vi "PAN_sendSchedCmd.vi"(6 "timeout in ms (5000)":i32=5000, 8 "error in (no error)":errorcluster, 10 "command":string) -> (0 "error out":errorcluster, 2 "response":string)   [LabVIEW 2016]
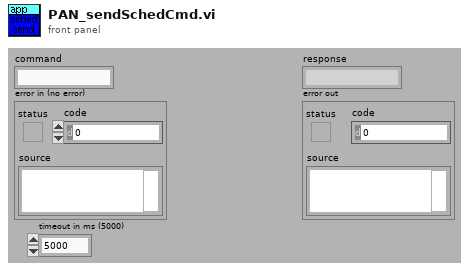
[diagram p1: front panel]
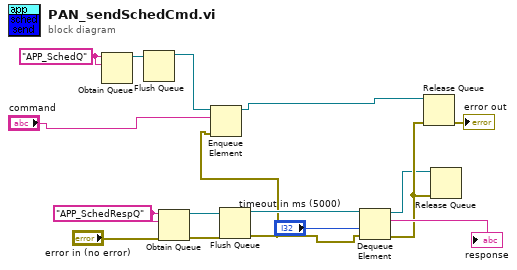
[diagram p0: block diagram]
diagram:
  w15 = "APP_SchedRespQ" ("name (unnamed)")
  w16 = "APP_SchedQ" ("name (unnamed)")
  n1 = Obtain Queue(name (unnamed)=w16, element data type=w16) -> (queue out=w10:refnum<queue>)  [unwired: 3 in, 2 out]
  n2 = Flush Queue(queue=w10) -> (queue out=w9:refnum<queue>)  [unwired: 1 in, 2 out]
  n3 = Obtain Queue(name (unnamed)=w15, element data type=w15, error in (no error)="error in (no error)") -> (queue out=w8:refnum<queue>, error out=w7:errorcluster)  [unwired: 2 in, 1 out]
  n4 = Flush Queue(queue=w8, error in (no error)=w7) -> (queue out=w6:refnum<queue>, error out=w5:errorcluster)  [unwired: 1 out]
  n5 = Enqueue Element(queue=w9, element="command", error in (no error)=w5) -> (queue out=w11:refnum<queue>)  [unwired: 3 out]
  n6 = Dequeue Element(queue=w6, timeout in ms (-1)="timeout in ms (5000)", error in (no error)=w5) -> (queue out=w12:refnum<queue>, element=→"response":string, error out=w13:errorcluster)  [unwired: 1 out]
  n7 = Release Queue(queue=w11, error in (no error)=w13) -> (error out=→"error out":errorcluster)  [unwired: 3 out]
  n8 = Release Queue(queue=w12, error in (no error)=w13) -> ()  [unwired: 4 out]
